vi "Unpack for gRPC.vi"(8 "error in":errorcluster, 9 "configuration / results":enum16{"Configuration", "Results"}(ring), 10 "any":T1, 11 "measurement plugin in":refnum<class "CAN-LIN Raw Bus Capture.lvclass">) -> (0 "error out":errorcluster, 2 "data value":variant, 3 "measurement plugin out":refnum<class "CAN-LIN Raw Bus Capture.lvclass">)   [LabVIEW 2025, in "CAN-LIN Raw Bus Capture.lvclass"]
uses:
  CAN-LIN Raw Bus Capture.lvclass
  <vilib>/gRPC/LabVIEW gRPC Library/Shared/Any.ctl
  Measurement Configuration.ctl
  CAN-LIN Raw Bus Capture UI/Toggle.ctl
  Measurement Results.ctl
  a521b266-ce99-437c-923d-067dcf1e07fd.vi
  3ecd018e-d556-4cbc-bc60-c4ba57204520.vi
  <vilib>/gRPC/LabVIEW gRPC Library/Server API/Translate Protobuf Error.vi
  <vilib>/AdvancedString/1D String Array to Delimited String.vi
  <vilib>/gRPC/LabVIEW gRPC Library/Server API/Server/Get Server DLL Path.vi
  CAN-LIN Raw Bus Capture.lvclass/CAN-LIN Raw Bus Capture.ctl
  <vilib>/Plug-In SDKs/Measurements/Measurement Plugin Service/Measurement Plugin Service.lvclass
  <vilib>/gRPC/LabVIEW gRPC Library/grpc-lvsupport-release.lvlib
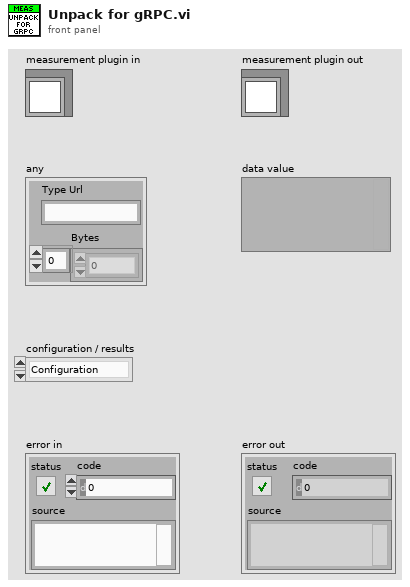
[diagram p1: front panel]
types:
  T1 = typedef "grpc-lvsupport-release.lvlib/Any.ctl" = cluster{"Type Url":string, "Bytes":u8[]}
  T2 = typedef "grpc-lvsupport-release.lvlib/grpcId.ctl" = u64
  T3 = typedef "CAN-LIN Raw Bus Capture.lvclass/Measurement Configuration.ctl" = cluster{"INTERFACE NAME CAN":refnum<k21>, "Termination CAN":T4, "FD Baudrate":u32, "Baudrate":u32, "FD ISO Mode":enum32{"ISO", "Legacy ISO", "Non-ISO"}, "IO Mode":enum32{"CAN", "CAN FD", "CAN FD + BRS"}, "SortByID":bool, "Filter":string, "INTERFACE NAME LIN":refnum<k21>, "Termination LIN":T4, "Can Interface":string}
  T4 = typedef "Toggle.ctl" = bool
  T5 = typedef "CAN-LIN Raw Bus Capture.lvclass/Measurement Results.ctl" = cluster{"CAN Bus Info":string, "Message Buffer":string[][]}
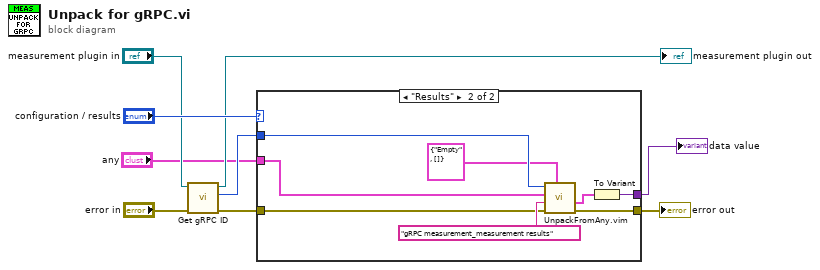
[diagram p0: block diagram]
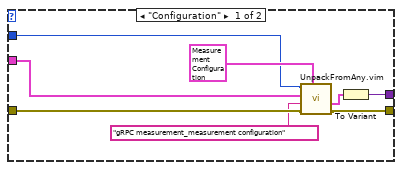
[diagram p2: hidden frame]
diagram:
  n1 = call <vilib>:"Get gRPC ID.vi"("error in"="error in", "measurement plugin service in"="measurement plugin in") -> ("error out"=w6:errorcluster, "gRPC ID"=w3:T2, "measurement plugin service out"=→"measurement plugin out":refnum<class "CAN-LIN Raw Bus Capture.lvclass">)  [unwired: 7 in]
  n2 = case shown="\"Results\"" "configuration / results" {
    tunnel: w6 -> [w15 w19]
    tunnel: "any" -> [w10 w18]
    tunnel: w3 -> [w12 w22]
    tunnel: [w16 w23] -> w9
    tunnel: [w17 w25] -> w1
    frame "Configuration" {
      n3 = call "UnpackFromAny.vim"("Data Type"=T3 {"INTERFACE NAME CAN"="", "Termination CAN"=FALSE, "FD Baudrate"=32, "Baudrate"=64, "FD ISO Mode"=enum."ISO", "IO Mode"=enum."CAN", "SortByID"=FALSE, "Filter"="", "INTERFACE NAME LIN"="", "Termination LIN"=FALSE, "Can Interface"=""} ("Measurement Configuration"), "error in"=w15, "Message Type"="gRPC measurement_measurement configuration", "Any"=w10, "gRPCid in"=w12) -> ("error out"=w16:errorcluster, "Unpacked Value"=w14:T3)  [unwired: 4 in, 1 out]
      n4 = To Variant(anything=w14) -> (Variant=w17:variant)
    }
    frame "Results" {
      n5 = call "UnpackFromAny.vim"("Data Type"=T5 {"CAN Bus Info"="Empty", "Message Buffer"=[]} ("Measurement Results"), "error in"=w19, "Message Type"="gRPC measurement_measurement results", "Any"=w18, "gRPCid in"=w22) -> ("error out"=w23:errorcluster, "Unpacked Value"=w24:T5)  [unwired: 4 in, 1 out]
      n6 = To Variant(anything=w24) -> (Variant=w25:variant)
    }
  }
  "error out" <- w9
  "data value" <- w1
